vi "Add Unique Parent.vi"(8 "error in":errorcluster, 10 "String":string, 11 "Tree Refnum in":refnum<vi>) -> (0 "error out":errorcluster, 3 "Tree Refnum out":refnum<vi>)   [LabVIEW 2019, in "Configuration.lvlib" / "Configuration.lvclass"]
uses:
  Configuration.lvclass
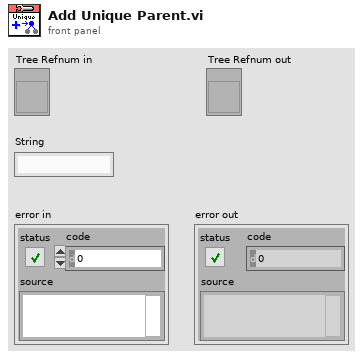
[diagram p1: front panel]
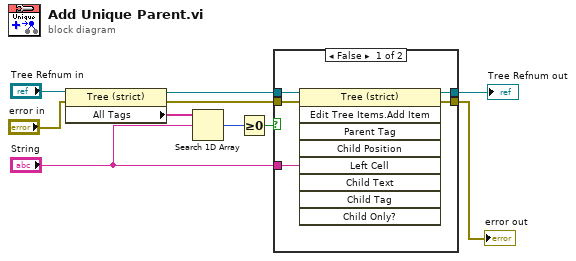
[diagram p0: block diagram]
diagram:
  n1 = property class="Tree (strict)"(reference="Tree Refnum in", error in="error in") -> (reference out=w9:refnum<vi>, error out=w2:errorcluster, "All Tags"=w7:string[])
  n2 = Search 1D Array(1D array=w7, element="String") -> (index of element=w5:i32)  [unwired: 1 in]
  n3 = Greater Or Equal To 0?(x=w5) -> (x >= 0?=w4:bool)
  n4 = case shown="False" w4 {
    tunnel: w9 -> [w15 w17]
    tunnel: [w14 w17] -> w8
    tunnel: "String" -> [w13 _]
    tunnel: w2 -> [w12 w16]
    tunnel: [w11 w16] -> w1
    frame False {
      n5 = invoke class="Tree (strict)" method="Edit Tree Items.Add Item"(reference=w15, error in=w12, "Left Cell"=w13) -> (reference out=w14:refnum<vi>, error out=w11:errorcluster)  [unwired: 6 in, 7 out]
    }
    frame True {
    }
  }
  "error out" <- w1
  "Tree Refnum out" <- w8
